vi "GetMultiBotIDs.vi"(8 "error in (no error)":errorcluster, 11 "manifest file":path) -> (0 "error out":errorcluster, 3 "Array":T1[](array[typedef]))   [LabVIEW 2014]
uses:
  simulation/SimulationIDs.ctl
  <vilib>/Robotics/Utilities/Generate Error.vi
  <vilib>/Robotics/Simulator/Interface/Simulator Configuration/Load Manifest File String.vi
  <vilib>/Robotics/Simulator/Utility/Resources Dealing/Extend Engine Resource Filepath.vi
  <vilib>/Utility/error.llb/Simple Error Handler.vi
  <vilib>/Robotics/Simulator/Engine/ODESimulator_Engine.lvclass
  <vilib>/Robotics/Simulator/Robot Classes/Base/ODESimulator_Base_Robot.lvclass
  <vilib>/Robotics/Simulator/Robot Factory/Sensor/Base/ODESimulator_Base_Sensor.lvclass
  <vilib>/Robotics/Simulator/Robot Factory/Motor/ODESimulator_Motor.lvclass
  <vilib>/robotics/Simulator/NI_Robotics_Simulator.lvlib
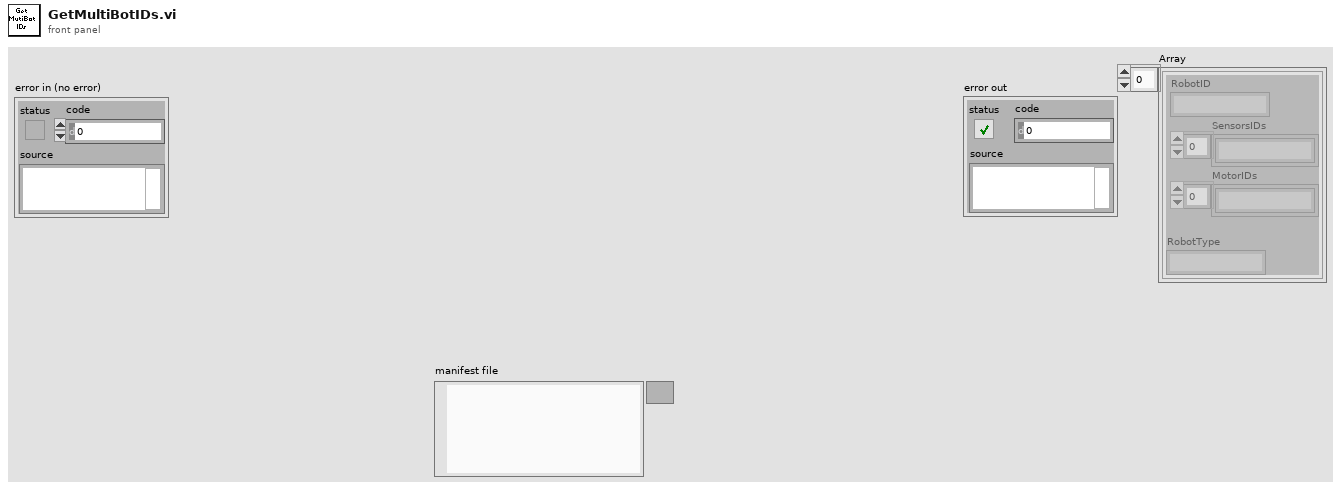
[diagram p1: front panel]
types:
  T1 = typedef "SimulationIDs.ctl" = cluster{"RobotID":string, "SensorsIDs":string[], "MotorIDs":string[], "RobotType":string}
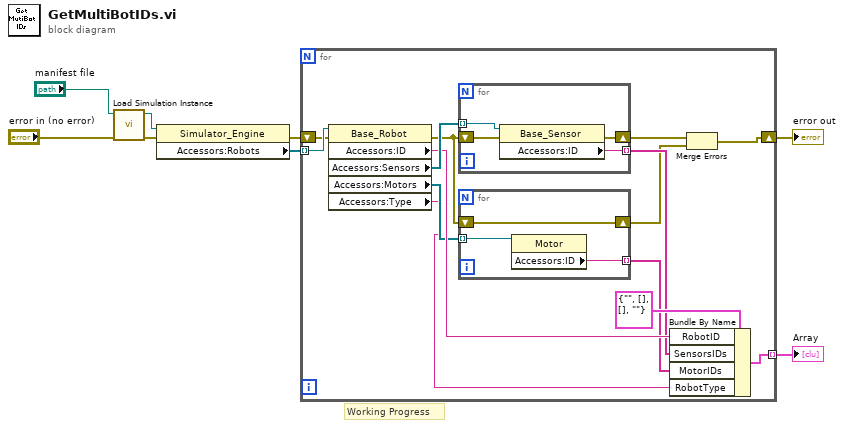
[diagram p0: block diagram]
diagram:
  # "Working Progress"
  n1 = call <vilib>:"Load Simulation Instance.vi"("error in (no error)"="error in (no error)", "manifest file"="manifest file") -> ("error out"=w5:errorcluster, "simulation instance"=w7:refnum<class "ODESimulator_Engine.lvclass">)  [unwired: 8 in]
  n2 = property class="Simulator_Engine"(reference=w7, error in=w5) -> (error out=w4:errorcluster, "Accessors:Robots"=w6:refnum<class "ODESimulator_Base_Robot.lvclass">[])  [unwired: 1 out]
  n3 = for {
    tunnel: w6 -> [w22] mode=indexing
    tunnel: [w15] -> w1 mode=indexing
    shift-right: [w10] -> w3
    shift-left: w4 -> [w14]
    n4 = property class="Base_Robot"(reference=w22, error in=w14) -> (error out=w13:errorcluster, "Accessors:ID"=w19:string, "Accessors:Sensors"=w21:refnum<class "ODESimulator_Base_Sensor.lvclass">[], "Accessors:Motors"=w17:refnum<class "ODESimulator_Motor.lvclass">[], "Accessors:Type"=w9:string)  [unwired: 1 out]
    n5 = for {
      tunnel: w21 -> [w29] mode=indexing
      tunnel: [w28] -> w18 mode=indexing
      shift-right: [w26] -> w12
      shift-left: w13 -> [w27]
      n6 = property class="Base_Sensor"(reference=w29, error in=w27) -> (error out=w26:errorcluster, "Accessors:ID"=w28:string)  [unwired: 1 out]
    }
    n7 = for {
      tunnel: w17 -> [w25] mode=indexing
      tunnel: [w24] -> w16 mode=indexing
      shift-right: [w23] -> w11
      shift-left: w13 -> [w23]
      n8 = property class="Motor"(reference=w25) -> ("Accessors:ID"=w24:string)  [unwired: 1 in, 2 out]
    }
    n9 = Bundle By Name(cluster=T1 {"RobotID"="", "SensorsIDs"=[], "MotorIDs"=[], "RobotType"=""} ("RoboSimIDs"), "RobotID"=w19, "SensorsIDs"=w18, "MotorIDs"=w16, "RobotType"=w9) -> (w15:T1)
    n10 = Merge Errors(w12, w11) -> (w10:errorcluster)
  }
  "error out" <- w3
  "Array" <- w1
